vi "Express Single Tone Informat.vi"(5 "search (+/- % of fund.)":dbl=5.0 format="%0.2p", 6 "approx freq. (optional)":dbl=-1.0 format="%0.2p", 7 "export signals":T1(ring)=enum."detected signal", 8 "time signal in":waveform(dbl)[](array[waveform])) -> (0 "exported spectrum":waveform(dbl)[](graph), 1 "detected phase (deg)":waveform(dbl)[](graph), 2 "detected amplitude":waveform(dbl)[](graph), 3 "detected frequency":waveform(dbl)[](graph), 4 "exported time signal":waveform(dbl)[](graph))   [LabVIEW 2017]
uses:
  <vilib>/measure/matone.llb/Extract Single Tone Information 1 Chan.vi
  <vilib>/measure/NI_MAPro.lvlib
panel:
  out "Array 3":dbl[](array[numeric]) format="%0.2f"
  out "Array 2":dbl[](array[numeric]) format="%0.2f"
  out "Array":dbl[](array[numeric]) format="%0.2f"
  # "Extract Single Tone\nInformation"
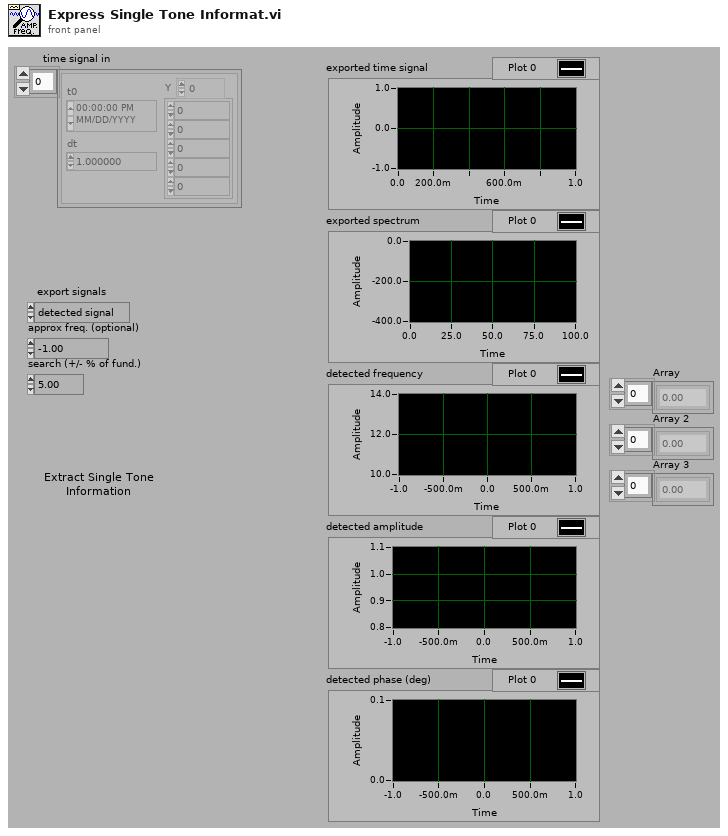
[diagram p1: front panel]
types:
  T1 = enum16{"none", "input signal", "detected signal", "residual signal"}
  T2 = cluster{"exported time signal":waveform(dbl), "exported spectrum (dB)":cluster{"f0":dbl, "df":dbl, "dB Spectrum (Hann)":dbl[]}}
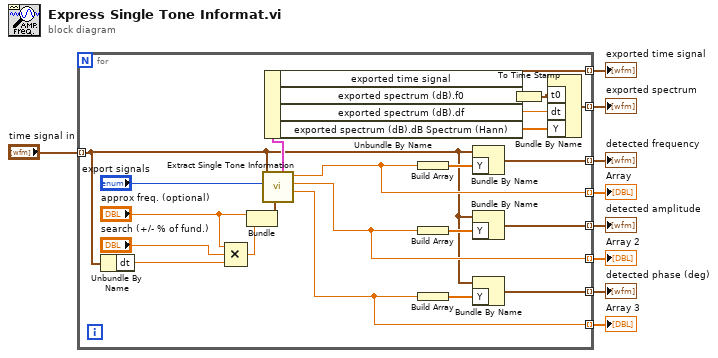
[diagram p0: block diagram]
diagram:
  n1 = for {
    tunnel: "time signal in" -> [w14] mode=indexing
    tunnel: [w30] -> w8 mode=indexing
    tunnel: [w26] -> w4 mode=indexing
    tunnel: [w21] -> w7 mode=indexing
    tunnel: [w20] -> w6 mode=indexing
    tunnel: [w19] -> w5 mode=indexing
    tunnel: [w18] -> w3 mode=indexing
    tunnel: [w17] -> w2 mode=indexing
    tunnel: [w16] -> w1 mode=indexing
    n2 = Unbundle By Name(w14) -> ("dt"=w15:dbl)
    n3 = Compound Arithmetic op=MULTIPLY("approx freq. (optional)", "search (+/- % of fund.)", w15) -> (w11:dbl)
    n4 = Bundle("approx freq. (optional)"="approx freq. (optional)", w11) -> (w25:cluster{"approx freq. (optional)":dbl, dbl})  [unwired: 1 in]
    n5 = call-poly <vilib>:"Extract Single Tone Information.vi"("advanced search"=w25, "export mode"="export signals", "time signal in"=w14) -> ("detected phase (deg)"=w16:dbl, "detected amplitude"=w17:dbl, "detected frequency"=w18:dbl, "exported signals"=w31:T2)  [unwired: 3 in, 2 out]
    n6 = Unbundle By Name(w31) -> ("exported time signal"=w30:waveform(dbl), "exported spectrum (dB).f0"=w29:dbl, "exported spectrum (dB).df"=w28:dbl, "exported spectrum (dB).dB Spectrum (Hann)"=w27:dbl[])
    n7 = Build Array(w18) -> (w24:dbl[])
    n8 = Build Array(w17) -> (w23:dbl[])
    n9 = Build Array(w16) -> (w22:dbl[])
    n10 = Bundle By Name(cluster=w14, "Y"=w24) -> (w21:waveform(dbl))
    n11 = Bundle By Name(cluster=w14, "Y"=w23) -> (w20:waveform(dbl))
    n12 = Bundle By Name(cluster=w14, "Y"=w22) -> (w19:waveform(dbl))
    n13 = To Time Stamp(1:w29) -> (0:w10:timestamp)
    n14 = Bundle By Name("t0"=w10, "dt"=w28, "Y"=w27) -> (w26:waveform(dbl))  [unwired: 1 in]
  }
  "exported time signal" <- w8
  "exported spectrum" <- w4
  "detected frequency" <- w7
  "detected amplitude" <- w6
  "detected phase (deg)" <- w5
  "Array" <- w3
  "Array 2" <- w2
  "Array 3" <- w1
